vi "Get String Entries.vi"(8 "error in (no error)":errorcluster, 11 "Results in":refnum<class "Results.lvclass">) -> (0 "error out":errorcluster, 2 "String Entries":T1[](array[typedef]), 3 "Results out":refnum<class "Results.lvclass">)   [LabVIEW 2020, in "Tester.lvlib" / "Results.lvclass"]
uses:
  Results.lvclass
  String Entry.ctl
  Results.lvclass/Results.ctl
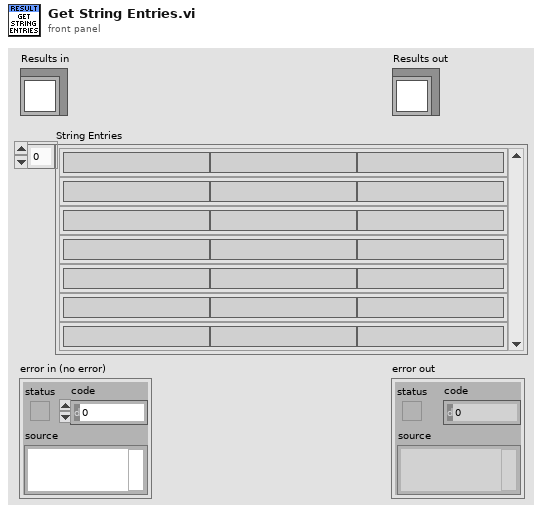
[diagram p1: front panel]
types:
  T1 = typedef "Tester.lvlib/Results.lvclass/String Entry.ctl" = cluster{"Name":string, "Value":string, "Result":string}
  T2 = typedef "Tester.lvlib/Results.lvclass/Results Ref.ctl" = cluster{"Entries":T3[], "Overall Result":T4}
  T3 = typedef "Tester.lvlib/Results.lvclass/Entry.ctl" = cluster{"Name":string, "Value":variant, "Result":T4}
  T4 = typedef "Tester.lvlib/Results.lvclass/Result.ctl" = enum16{"No Result", "Pass", "Fail", "Error", "Abort"}
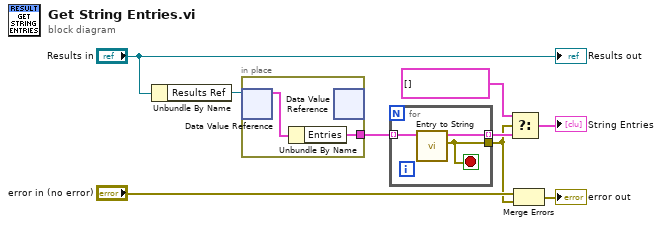
[diagram p0: block diagram]
diagram:
  n1 = Unbundle By Name("Results in") -> ("Results Ref"=w8:refnum<data-value>)
  n2 = in-place {
    in-place-border: [w10] -> w6
    n3 = in-place-dvr #1(w8) -> (w11:T2)  [unwired: 1 out]
    n4 = Unbundle By Name(w11) -> ("Entries"=w10:T3[])
    n5 = in-place-dvr #1() -> ()  [unwired: 1 in, 2 out]
  }
  n6 = for {
    tunnel: w6 -> [w14] mode=indexing
    tunnel: [w13] -> w5 mode=indexing
    tunnel: [w12] -> w1
    stop <- w12 stop-if-true
    n7 = call "Entry to String.vi"("Entry"=w14) -> ("error out"=w12:errorcluster, "String Entry"=w13:T1)  [unwired: 9 in]
  }
  n8 = Select(t=T1[] [], s=w1, f=w5) -> (s? t:f=→"String Entries":T1[])
  n9 = Merge Errors("error in (no error)", w1) -> (→"error out":errorcluster)
  "Results out" <- "Results in"
